vi "Read Sideways Drive State.vi"(8 "error in (no error)":errorcluster, 11 "Sideways Drive in":refnum<class "Sideways Drive.lvclass">) -> (0 "error out":errorcluster, 2 "Sideways Drive State":T1 {"Sideways Drive Power" min=-1.0 max=1.0 scale=-1.0..1.0}, 3 "Sideways Drive out":refnum<class "Sideways Drive.lvclass">)   [LabVIEW 2014, in "Sideways Drive.lvlib" / "Sideways Drive.lvclass"]
uses:
  Sideways Drive.lvclass
  Sideways Drive State.ctl
  Sideways Drive.lvclass/Sideways Drive.ctl
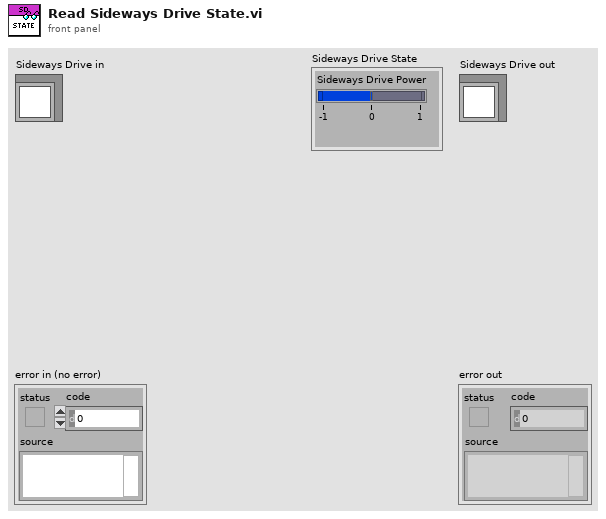
[diagram p1: front panel]
types:
  T1 = typedef "Sideways Drive.lvlib/Sideways Drive.lvclass/Sideways Drive State.ctl" = cluster{"Sideways Drive Power ":dbl}
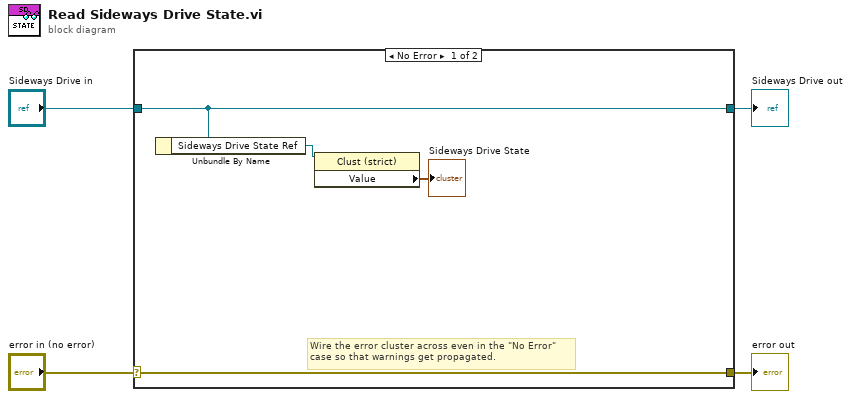
[diagram p0: block diagram]
diagram:
  n1 = case shown="No Error" "error in (no error)" {
    selector: "error in (no error)" -> [w8 w10]
    tunnel: [w8 w10] -> w3
    tunnel: [w7 w9] -> w1
    tunnel: "Sideways Drive in" -> [w7 w9]
    frame No Error {
      # "Wire the error cluster across even in the \"No Error\"\ncase so that warnings get propagated."
      n2 = Unbundle By Name(w7) -> ("Sideways Drive State Ref"=w6:refnum<vi>)
      n3 = property class="Clust (strict)"(reference=w6) -> ("Value"=→"Sideways Drive State":T1)  [unwired: 1 in, 2 out]
    }
    frame Error {
    }
  }
  "error out" <- w3
  "Sideways Drive out" <- w1
